vi "angle_LUT.vi"(1 "cell":i32) -> (0 "angle":dbl)   [LabVIEW 2015, in "PolyVIEW.lvclass"]
uses:
  PolyVIEW.lvclass
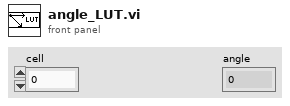
[diagram p1: front panel]
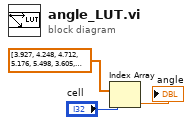
[diagram p0: block diagram]
diagram:
  n1 = Index Array(array=dbl[] [3.927, 4.248, 4.712, 5.176, 5.498, 3.605, 3.927, 4.712, 5.498, 5.82, 3.142, 3.142, nan, 0.0, 0.0, 2.678, 2.356, 1.571, 0.785, 0.464, 2.356, 2.034, 1.571, 1.107, 0.785], index="cell") -> (element=→"angle":dbl)
